vi "ExCascadeNframe128.vi"() -> ()   [LabVIEW 2010]
panel:
  in  "ADC Gain":u32
  out "ADC Speed (Khz)":u32
  in  "Avalanche Gain\nOnly valid for \nport 0":dbl format="%.2f"
  in  "ReadOut Port":u32 max=1 step=1
  in  "Trigger Edge":u32(ring)=1 items=["", "Positive (leading) edge", "Negative (falling) Edge"]
  in  "Trigger/Timing Mode":u32(ring)=1 items=["N/A", "FreeRun/Timed", "Single Trigger (PM only)", "Ext Sync/Strobed", "Bulb (PM only)", "Variable (PM only)", "Flash Mode (PM only)"]
  in  "Y End":u32=128 min=1 step=1
  in  "Y Start":u32=1 min=1 step=1
  in  "X Bin":u32=1 min=1 step=1
  in  "X End":u32=128 min=1 step=1
  in  "Y Bin":u32=1 min=1 step=1
  in  "X Start":u32=1 min=1 step=1
  in  "Number of Images":u32=2130 min=1 step=1
  in  "Temperature":dbl=-10.0 format="%.2f"
  in  "Exposure":dbl min=0.0 step=0.001 format="%.3f"
  out "error out":errorcluster
  in  "error in (no error)":errorcluster
  # "ExCascadeNframe128:\nThis example sets up the camera with a given ROI, and \ncollects into a file \"number of Images\"  set by user. The \nImages are also displayed.\nNote: not all cameras support nframe.\nThis also shows how to setup the Cascade for nframe"
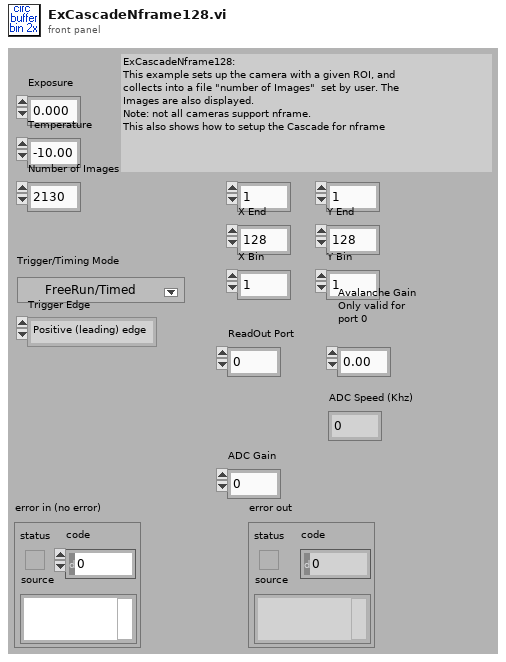
[diagram p1: front panel]
types:
  T1 = cluster{"X Start":u32, "X End":u32, "X Bin":u32, "Y Start":u32, "Y End":u32, "Y Bin":u32}
  T2 = cluster{"acquire focus mode":u32, "Exposure":dbl, "Number of Images":u32, "Software accumulation":u32}
  T3 = cluster{"Camera Handle":u32, "Pulser Handle":u32, "File Handle":u32, "Display Handle":u32, "Image Handle":u32}
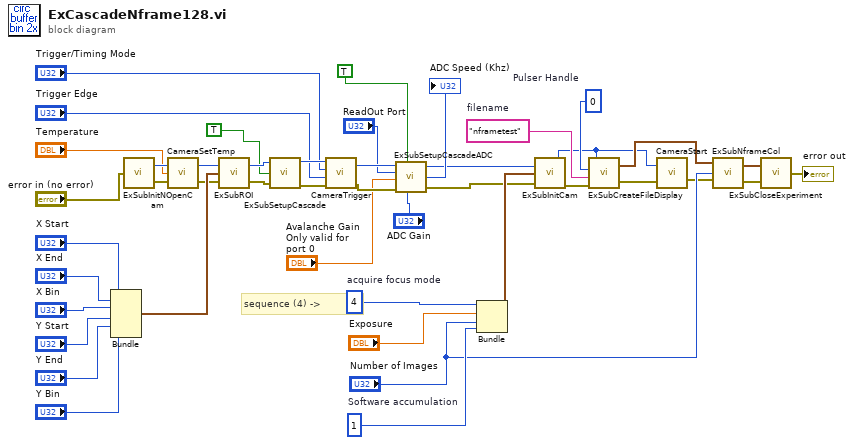
[diagram p0: block diagram]
diagram:
  w34 = u32 0  # Pulser Handle
  w36 = u32 4  # acquire focus mode
  w35 = u32 1  # Software accumulation
  w44 = "nframetest"  # filename
  # "sequence (4) ->"
  n1 = Bundle("X Start"="X Start", "X End"="X End", "X Bin"="X Bin", "Y Start"="Y Start", "Y End"="Y End", "Y Bin"="Y Bin") -> (w24:T1)  [unwired: 1 in]
  n2 = call "ExSubInitNOpenCam.vi"("error in (no error)"="error in (no error)") -> ("Camera Handle"=w19:u32, "error out"=w18:errorcluster)
  n3 = call <userlib>:"CameraSetTemp.vi"("error in (no error)"=w18, "Temperature"="Temperature", "Camera Handle"=w19) -> ("error out"=w16:errorcluster, "Camera Handle"=w17:u32)
  n4 = call "ExSubROI.vi"("error in (no error)"=w16, "ROI"=w24, "Camera Handle"=w17) -> ("error out"=w13:errorcluster, "Camera Handle"=w14:u32)
  n5 = call "ExSubSetupCascade.vi"("error in (no error)"=w13, "OverLap Mode"=TRUE, "Camera Handle"=w14) -> ("error out"=w37:errorcluster, "Camera Handle"=w38:u32)
  n6 = call <userlib>:"CameraTrigger.vi"("error in"=w37, "Trigger Edge"="Trigger Edge", "Timing Mode"="Trigger/Timing Mode", "Camera Handle"=w38) -> ("error out"=w9:errorcluster, "Camera Handle"=w10:u32)
  n7 = call "ExSubSetupCascadeADC.vi"("Camera Handle"=w10, "Fast ADC"=TRUE, "ReadOut Port"="ReadOut Port", "Avalanche Gain\nOnly valid for \nport 0"="Avalanche Gain\nOnly valid for \nport 0", "ADC Gain"="ADC Gain", "error in (no error)"=w9) -> ("Camera Handle"=w4:u32, "ADC Speed (Khz)"=→"ADC Speed (Khz)":u32, "error out"=w3:errorcluster)
  n8 = Bundle("acquire focus mode"=w36, "Exposure"="Exposure", "Number of Images"="Number of Images", "Software accumulation"=w35) -> (w41:T2)  [unwired: 1 in]
  n9 = call "ExSubInitCam.vi"("error in (no error)"=w3, "Camera Information"=w41, "Camera Handle"=w4) -> ("error out"=w40:errorcluster, "Camera Handle"=w20:u32)
  n10 = call "ExSubCreateFileDisplay.vi"("error in (no error)"=w40, "File and Display Name"=w44, "Pulser Handle"=w34, "Camera Handle"=w20) -> ("error out"=w23:errorcluster, "Handles Out"=w21:T3)
  n11 = call <userlib>:"CameraStart.vi"("error in"=w23, "Camera Handle"=w20) -> ("error out"=w22:errorcluster)  [unwired: 1 out]
  n12 = call "ExSubNframeCol.vi"("error in (no error)"=w22, "Number of Images"="Number of Images", "Handle Cluster"=w21) -> ("error out"=w32:errorcluster, "Handle Cluster"=w33:T3)
  n13 = call "ExSubCloseExperiment.vi"("error in (no error)"=w32, "Handles In"=w33) -> ("error out"=→"error out":errorcluster)
